vi "Recurse Sum of Last Diagonal.vi"(10 "Data":i64[](array[numeric]), 11 "Result In":i64) -> (3 "Result out":i64)   [LabVIEW 2020, in "Measurement.lvclass"]
uses:
  Measurement.lvclass
  Measurement.lvclass/Measurement.ctl
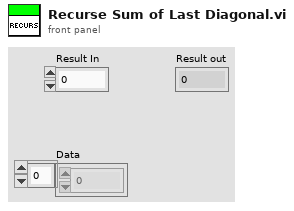
[diagram p1: front panel]
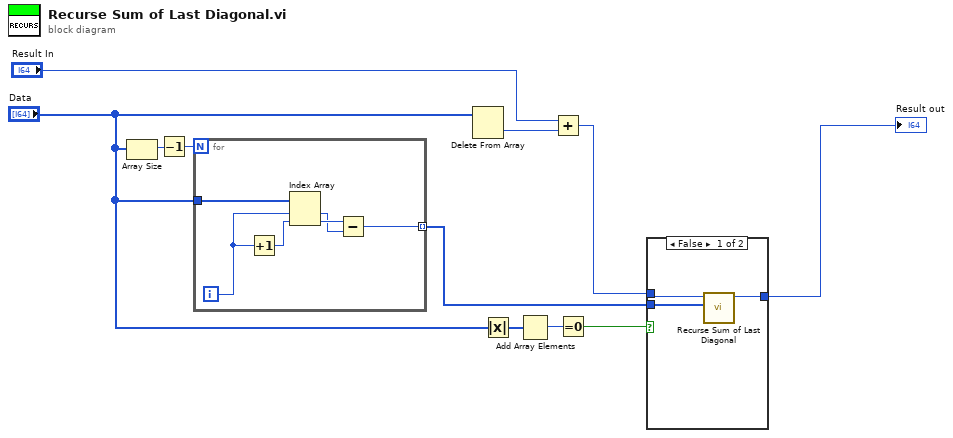
[diagram p0: block diagram]
diagram:
  n1 = Array Size(array="Data") -> (size(s)=w8:i32)
  n2 = Decrement(x=w8) -> (x-1=w9:i32)
  n3 = for {
    N: w9 -> [_]
    tunnel: "Data" -> [w17]
    tunnel: [w12] -> w4 mode=indexing
    i -> [w15]
    n4 = Increment(x=w15) -> (x+1=w16:i32)
    n5 = Index Array(array=w17, index #1=w15, index #2=w16) -> (element #1=w13:i64, element #2=w14:i64)
    n6 = Subtract(x=w14, y=w13) -> (x-y=w12:i64)
  }
  n7 = Delete From Array(array="Data") -> (deleted portion=w11:i64)  [unwired: 2 in, 1 out]
  n8 = Absolute Value(x="Data") -> (abs(x)=w1:i64[])
  n9 = Add Array Elements(numeric array=w1) -> (sum=w7:i64)
  n10 = Add(x="Result In", y=w11) -> (x+y=w5:i64)
  n11 = Equal To 0?(x=w7) -> (x = 0?=w6:bool)
  n12 = case shown="False" w6 {
    tunnel: w5 -> [w20 w21]
    tunnel: w4 -> [w19 _]
    tunnel: [w18 w21] -> w3
    frame False {
      n13 = call "Recurse Sum of Last Diagonal.vi"("Data"=w19, "Result In"=w20) -> ("Result out"=w18:i64)  [unwired: 9 in]
    }
    frame True {
    }
  }
  "Result out" <- w3
